vi "stop.vi"(8 "error in (no error)":errorcluster, 11 "Camera in":refnum<class "Camera.lvclass">) -> (0 "error out":errorcluster, 3 "Camera out":refnum<class "Camera.lvclass">)   [LabVIEW 2019, in "Camera.lvclass"]
doc: "Stops the current recording. In 'ring buffer' and 'fifo' mode, this function must be called\nby the user. In 'sequence' and 'sequence non blocking' mode, this function is automatically\ncalled when the number_of_images is reached."
uses:
  Camera.lvclass
  Camera.lvclass/Camera.ctl
  pco.recorder/Recorder.lvlib
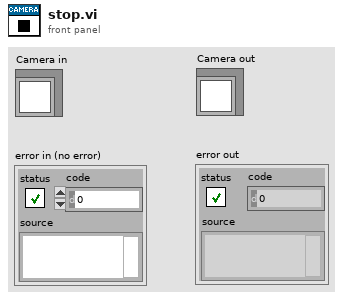
[diagram p1: front panel]
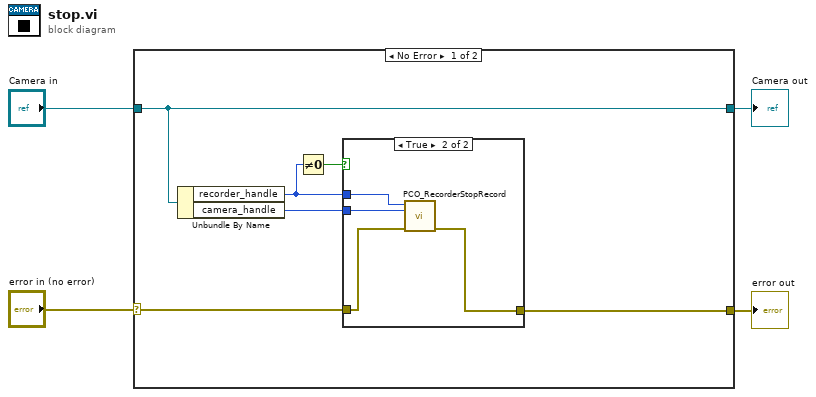
[diagram p0: block diagram]
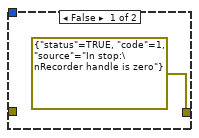
[diagram p2: hidden frame]
diagram:
  n1 = case shown="No Error" "error in (no error)" {
    selector: "error in (no error)" -> [w9 w17]
    tunnel: [w8 w17] -> w3
    tunnel: [w5 w16] -> w1
    tunnel: "Camera in" -> [w5 w16]
    frame No Error {
      n2 = Unbundle By Name(w5) -> ("recorder_handle"=w7:u64, "camera_handle"=w6:u64)
      n3 = Not Equal To 0?(x=w7) -> (x != 0?=w10:bool)
      n4 = case shown="True" w10 {
        tunnel: [errorcluster {"status"=TRUE, "code"=1, "source"="In stop:\nRecorder handle is zero"} ("error constant") w13] -> w8
        tunnel: w7 -> [_ w14]
        tunnel: w9 -> [_ w15]
        tunnel: w6 -> [_ w12]
        frame False {
        }
        frame True {
          n5 = call "PCO_RecorderStopRecord.vi"("error in (no error)"=w15, "phCam"=w12, "phRec"=w14) -> ("error out"=w13:errorcluster)  [unwired: 6 in, 2 out]
        }
      }
    }
    frame Error {
    }
  }
  "error out" <- w3
  "Camera out" <- w1
